vi "Test CAN Logger.vi"() -> ()   [LabVIEW 2014]
uses:
  <vilib>/RioEmbeddedCAN/RioEmbeddedCAN.llb/CANFrameControl.ctl
panel:
  out "index 2":i32
  in  "x":bool
  out "Array 2":T1[](array[typedef]) {"type" items=["CAN Data", "CAN Remote"]; "identifier" format="%.0x"}
  out "error out":errorcluster
  out "index":i32
  in  "baud rate (125000 bps)":u32=1000000
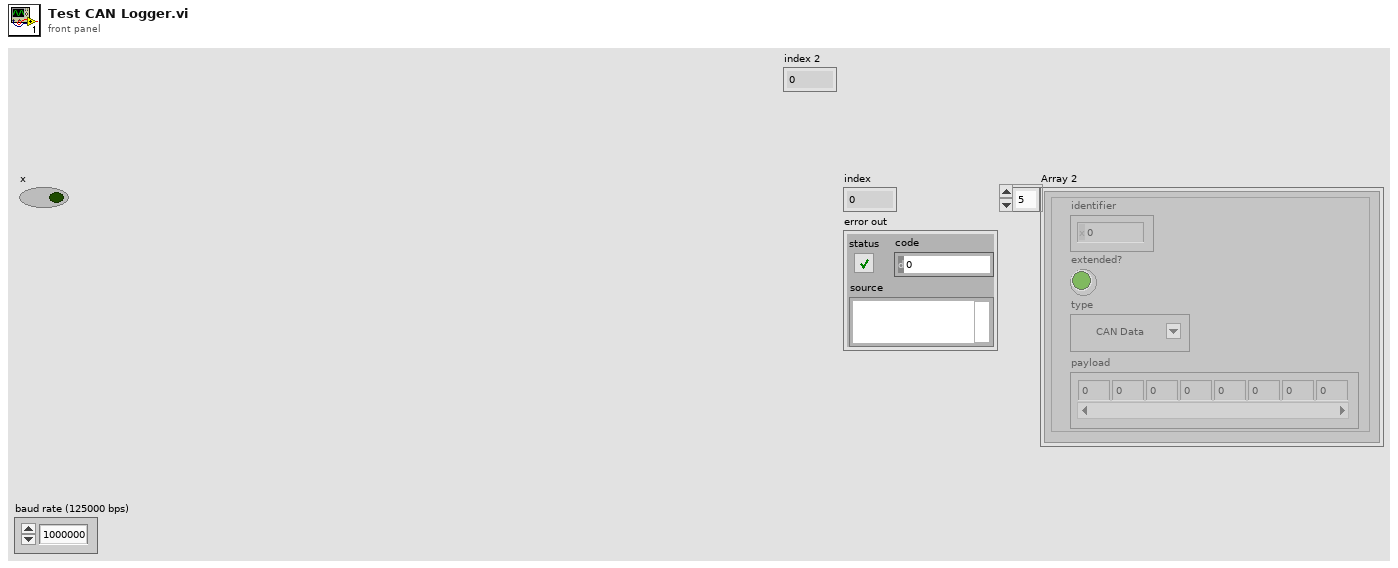
[diagram p1: front panel]
types:
  T1 = typedef "CANFrameControl.ctl" = cluster{"identifier":u32, "extended?":bool, "type":u8, "payload":u8[]}
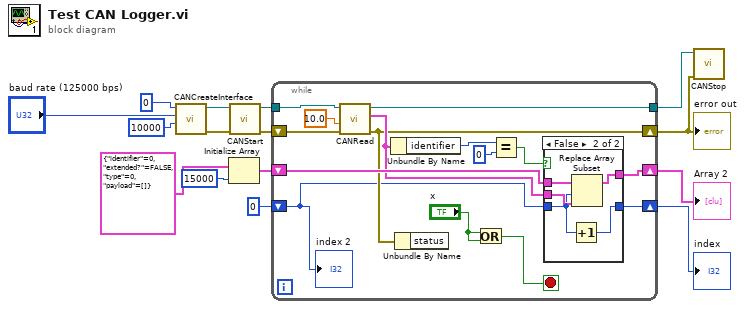
[diagram p0: block diagram]
diagram:
  n1 = call <vilib>:"CANCreateInterface.vi"("receive queue size (5)"=u32 10000, "baud rate (125000 bps)"="baud rate (125000 bps)", "interface index"=u32 0) -> ("error out"=w15:errorcluster, "interface object out"=w14:refnum<k20>)  [unwired: 7 in]
  n2 = Initialize Array(T1 {"identifier"=0, "extended?"=FALSE, "type"=0, "payload"=[]} ("CAN frame"), 15000 ("dimension size")) -> (w7:T1[])
  n3 = call <vilib>:"CANStart.vi"("error in (no error)"=w15, "interface object in"=w14) -> ("error out"=w4:errorcluster, "interface object out"=w13:refnum<k20>)  [unwired: 8 in]
  n4 = while {
    tunnel: w13 -> [w30]
    tunnel: [w29] -> w12
    shift-right: [w22] -> w1
    shift-left: w7 -> [w28]
    shift-right: [w23] -> w2
    shift-left: 0 ("index") -> [w16]
    shift-right: [w19] -> w11
    shift-left: w4 -> [w20]
    stop <- w18 stop-if-true
    n5 = call <vilib>:"CANRead.vi"("error in (no error)"=w20, "timeout (0 s)"=10.0, "interface object in"=w30) -> ("error out"=w19:errorcluster, "CAN frame"=w27:T1, "interface object out"=w29:refnum<k20>)  [unwired: 5 in, 1 out]
    n6 = Unbundle By Name(w27) -> ("identifier"=w26:u32)
    n7 = Unbundle By Name(w19) -> ()  [unwired: 1 out]
    n8 = Or(x="x", y="x") -> (x .or. y?=w18:bool)
    n9 = Equal?(x=w26, y=u32 0) -> (x = y?=w24:bool)
    n10 = case shown="False" w24 {
      tunnel: w28 -> [w32 w37]
      tunnel: [w32 w36] -> w22
      tunnel: w16 -> [w31 w34]
      tunnel: w27 -> [_ w35]
      tunnel: [w31 w33] -> w23
      frame True {
      }
      frame False {
        n11 = Increment(x=w34) -> (x+1=w33:i32)
        n12 = Replace Array Subset(array=w37, new element=w35, index=w34) -> (w36:T1[])
      }
    }
    "index 2" <- w16
  }
  "index" <- w2
  "error out" <- w11
  "Array 2" <- w1
  n13 = call <vilib>:"CANStop.vi"("error in (no error)"=w11, "interface object in"=w12) -> ()  [unwired: 8 in, 2 out]
